vi "temperature sweep -- read log.vi"() -> ()   [LabVIEW 2010]
uses:
  <vilib>/Analysis/6fits.llb/Curve Fitting Criteria.ctl
  <vilib>/regexp/Match Regular Expression.xnode
  <vilib>/Utility/file.llb/Read From Spreadsheet File (string).vi
  <vilib>/Analysis/3filter.llb/IIR Filter (DBL).vi
  <vilib>/Analysis/NI_AALPro.lvlib
  <vilib>/ptbypt/NI_PtbyPt.lvlib
  <vilib>/Analysis/NI_AALBase.lvlib
panel:
  in  "window (min)":dbl=1.0
  out "window 5":cluster{dbl[], dbl[]}[](graph)
  out "window 4":cluster{dbl[], dbl[]}[](graph)
  out "window 3":cluster{dbl[], dbl[]}[](graph)
  out "window 2":cluster{dbl[], dbl[]}[](graph)
  out "window":cluster{dbl[], dbl[]}[](graph)
  in  "Control ITC Log":path=path "C:/Data/GloveBox/Pu/239 Pu A/300K - 600K/Stability_081211.dat"
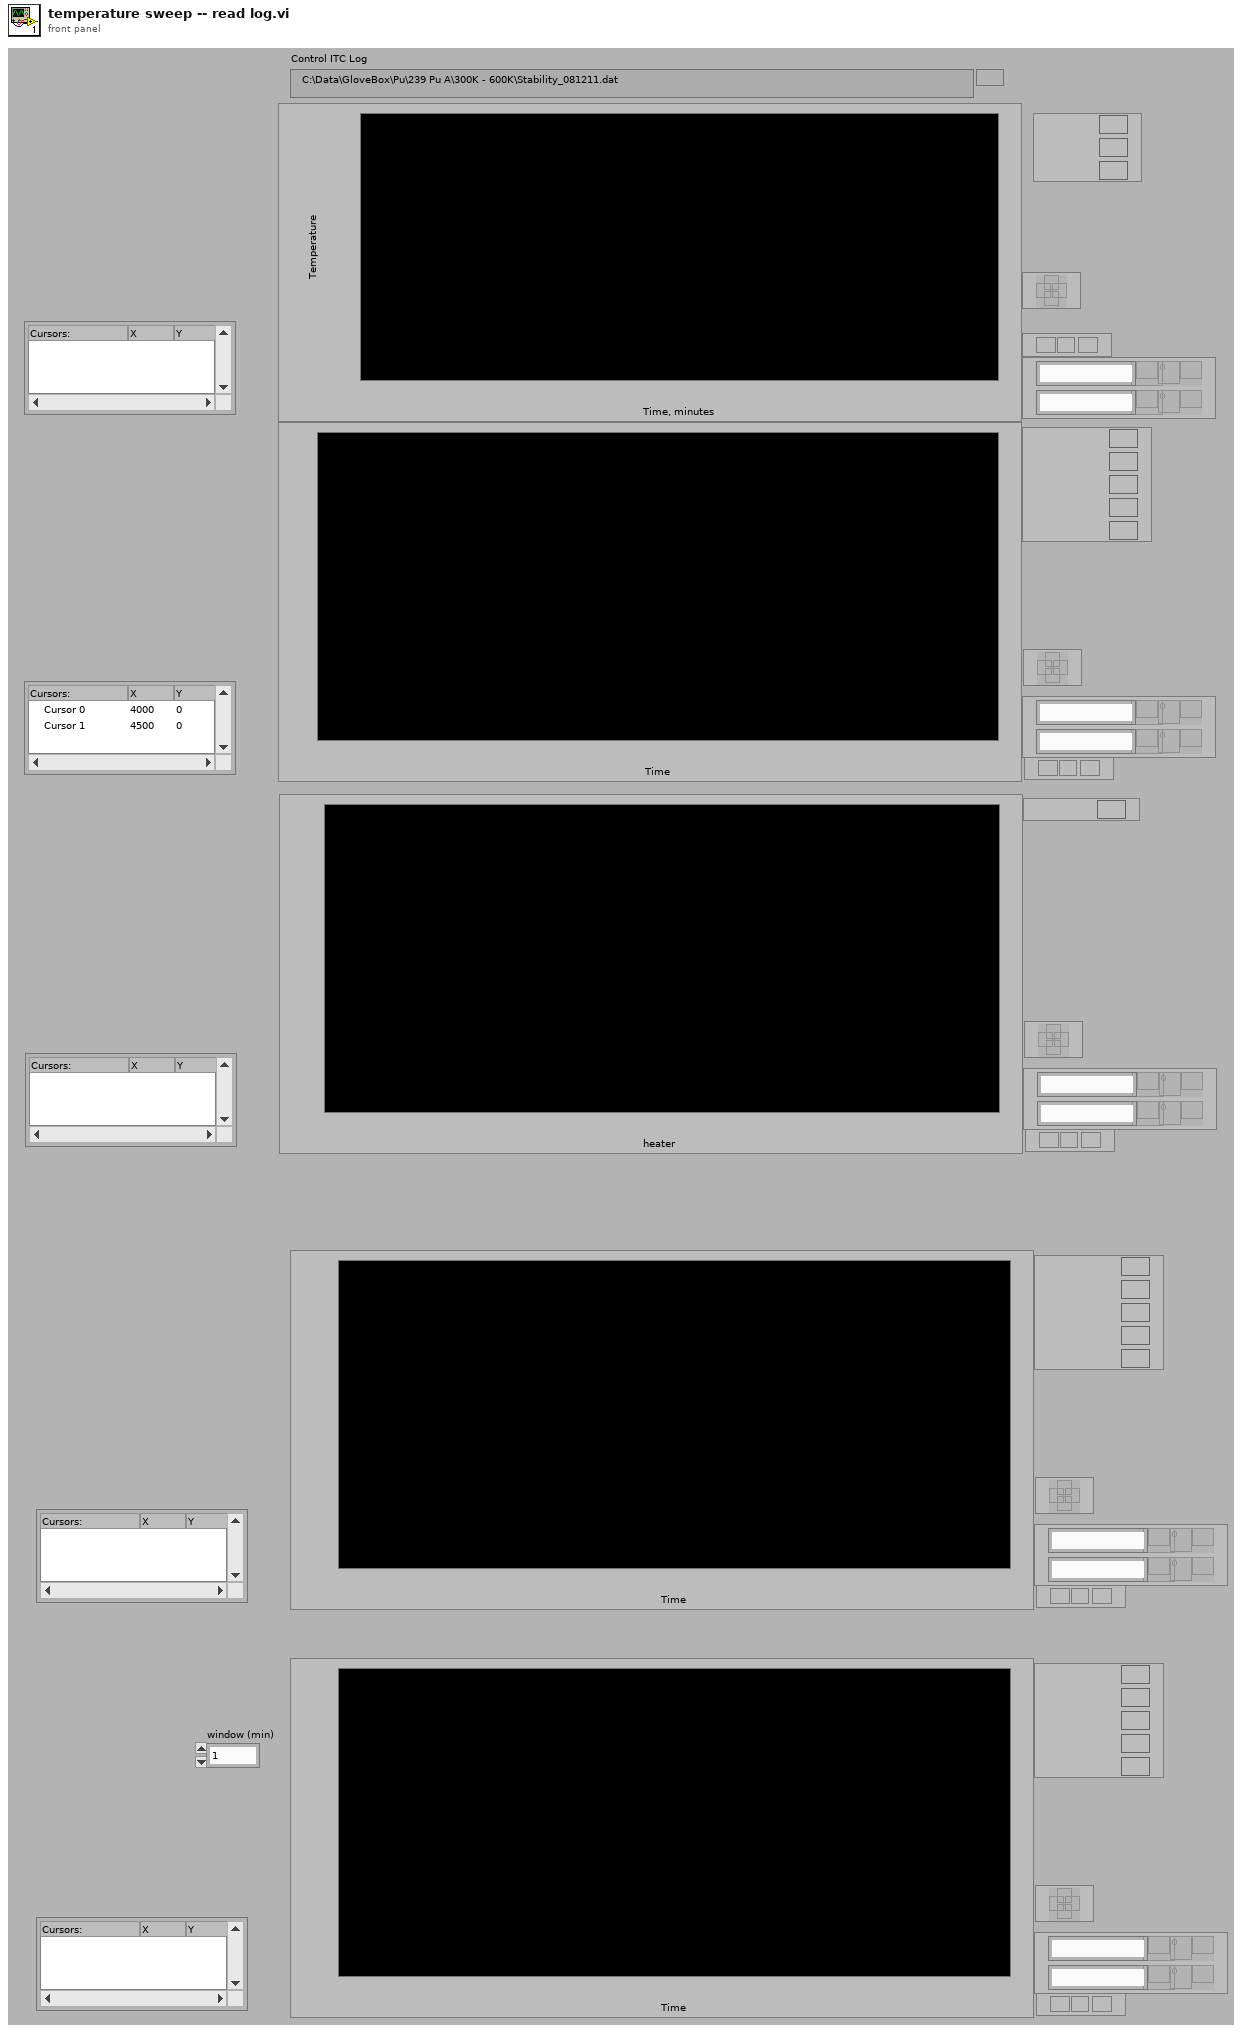
[diagram p1: front panel]
types:
  T1 = typedef "NI_AALPro.lvlib/Curve Fitting Criteria.ctl" = u16
  T2 = typedef "LVCursorListTypeDef.ctl" = cluster{"Name":string, "Color":u32, "Style":u8, "Point Style":u8, "Name Visible":bool, "Allow Drag":bool, "Cursor Mode":u32, "Plot":i32, "Index":i32, "Position":cluster{"X":dbl, "Y":dbl}, "X Scale":u32, "Y Scale":u32, "Watch Plots":i32[], "Watch All Plots":bool, "Plot Area":i32, "Label Offset":cluster{"X":dbl, "Y":dbl}}[]
  T3 = cluster{"omega out":dbl[], "whatever out":dbl[]}[]
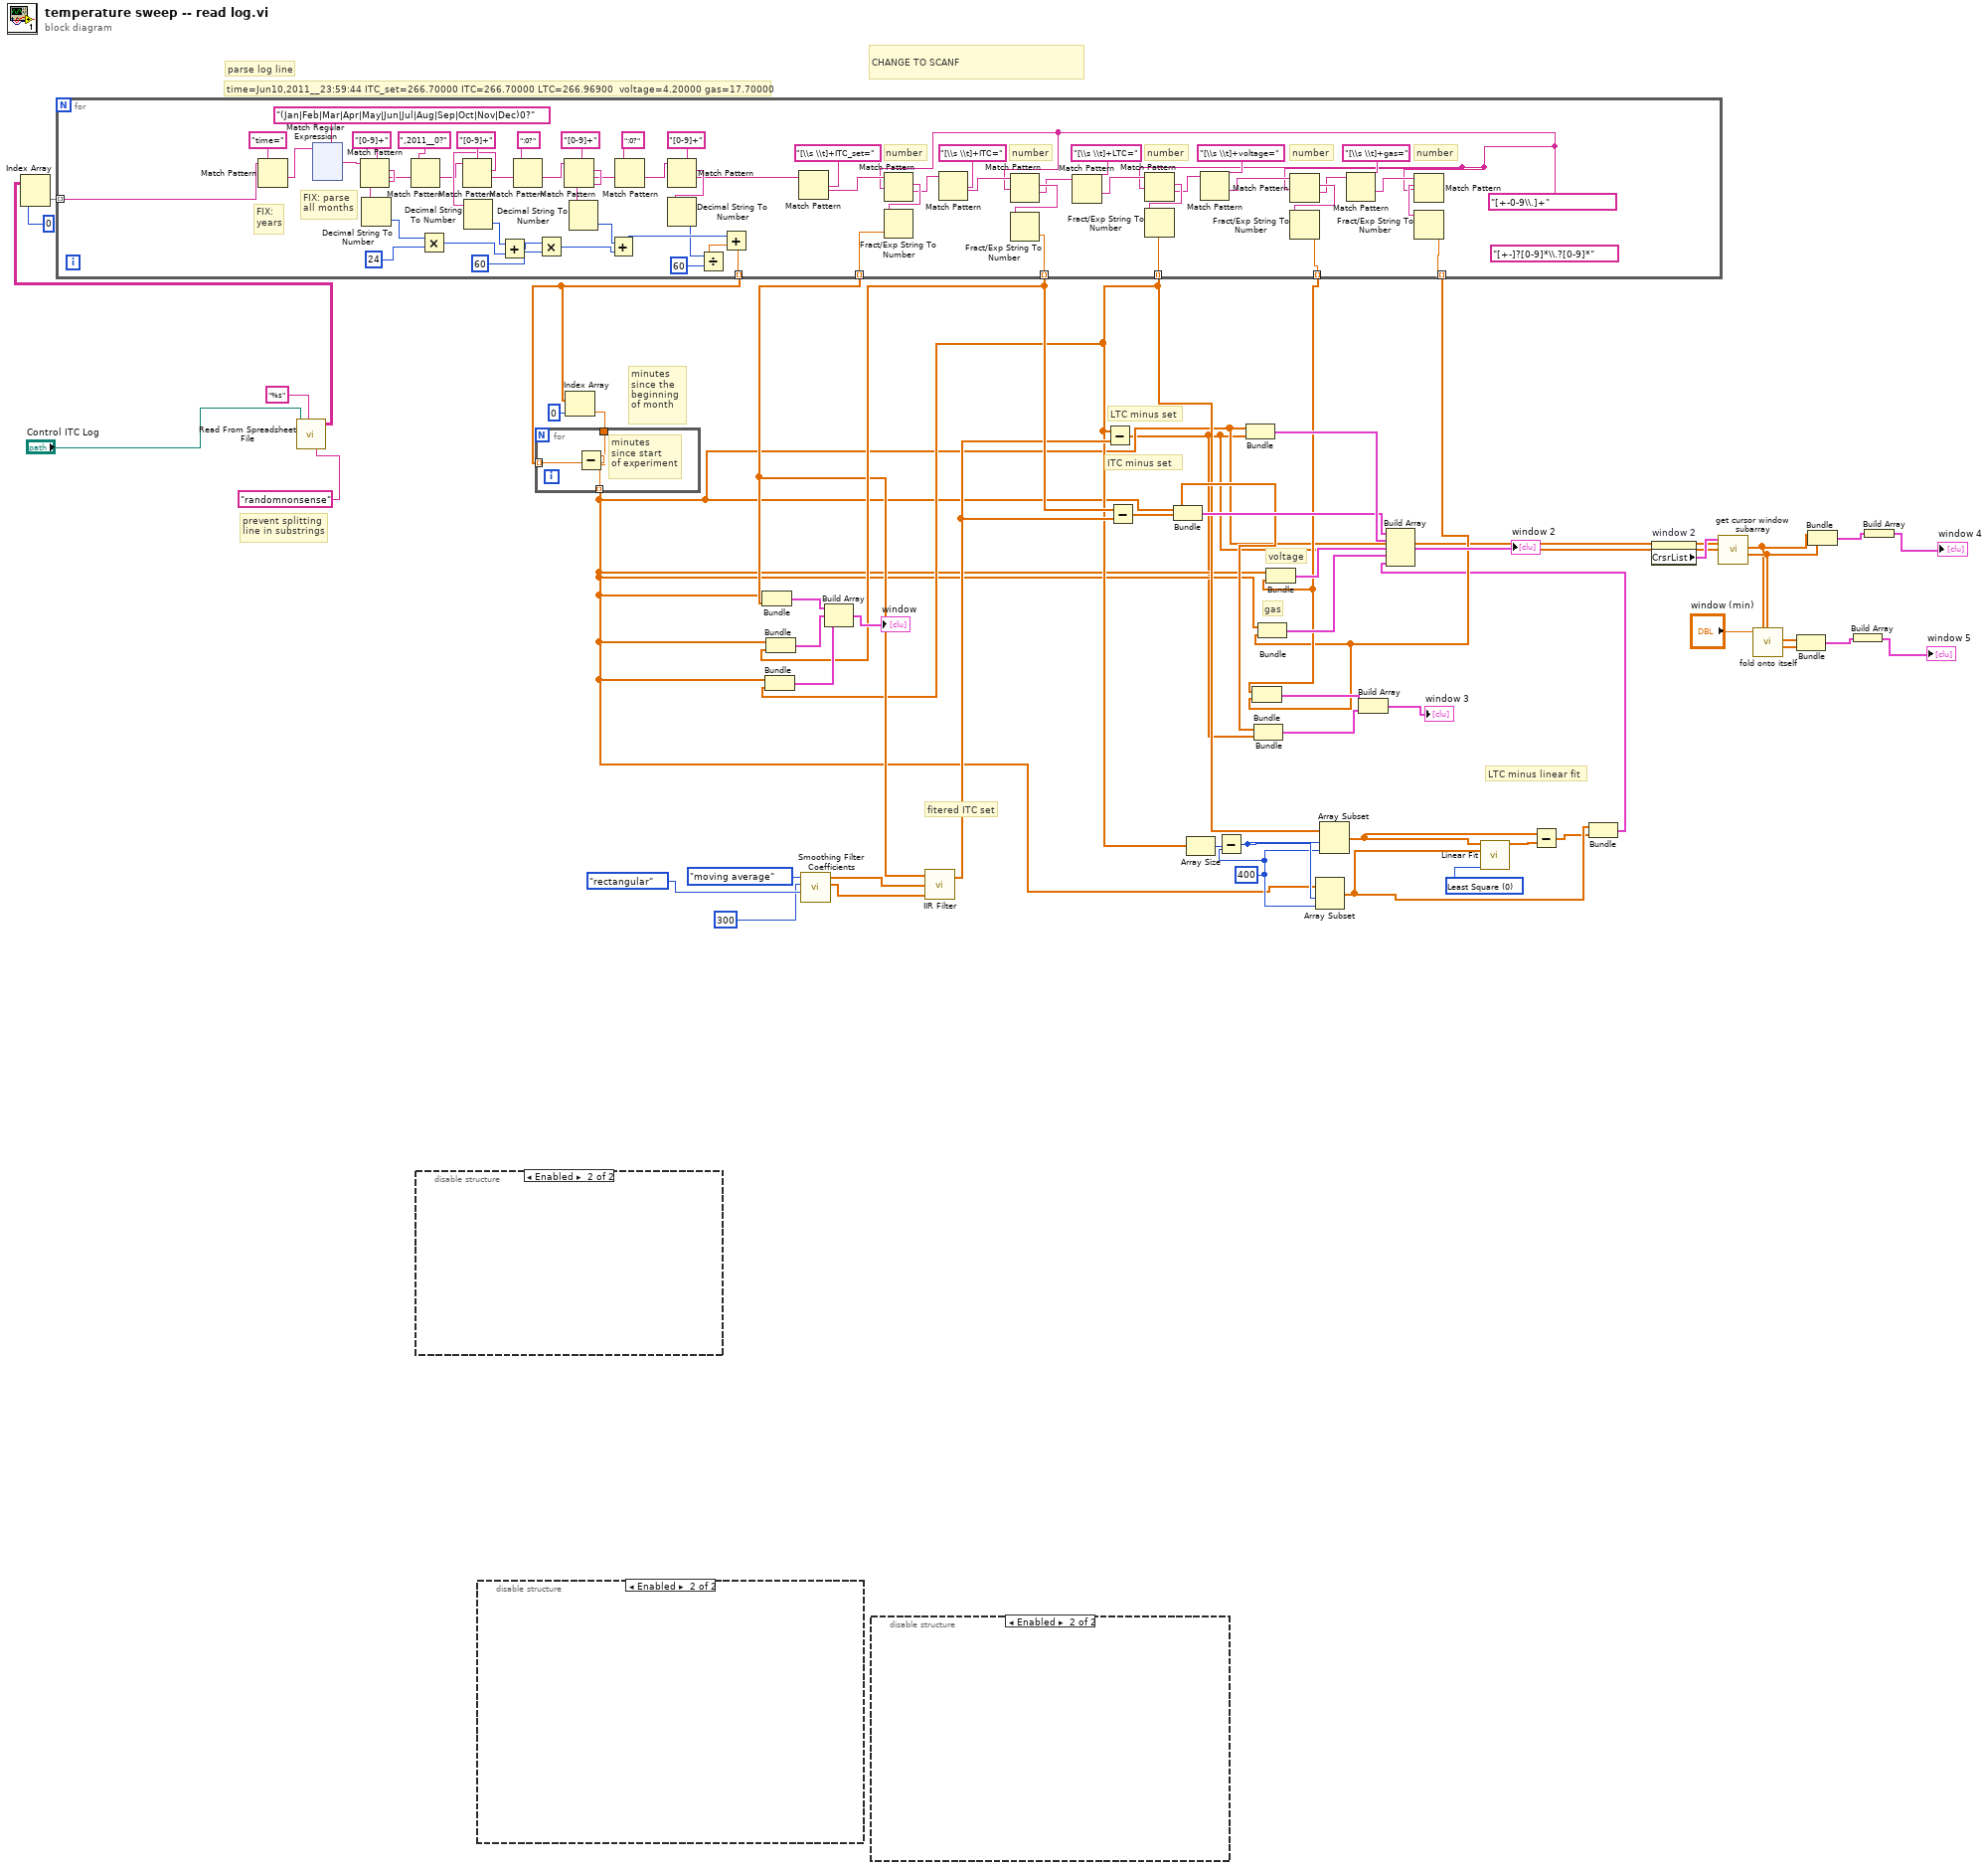
[diagram p0: block diagram]
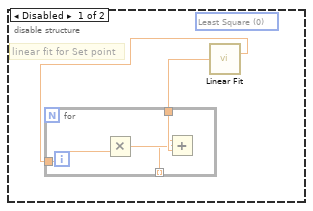
[diagram p2: hidden frame]
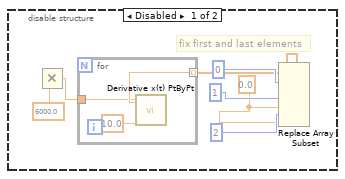
[diagram p3: hidden frame]
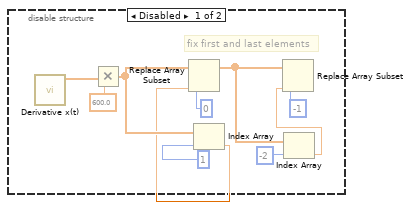
[diagram p4: hidden frame]
diagram:
  w18 = 400 ("length")
  w22 = T1 0 items=["Least Square", "Least Absolute Residual", "Bisquare"] ("method")
  # "fitered ITC set"
  # "CHANGE TO SCANF"
  # "LTC minus linear fit"
  # "minutes\nsince the\nbeginning \nof month"
  # "prevent splitting \nline in substrings"
  # "LTC minus set"
  # "gas"
  # "voltage"
  # "ITC minus set"
  # "parse log line"
  # "time=Jun10,2011__23:59:44\tITC_set=266.70000\tITC=266.70000\tLTC=266.96900\t\tvoltage=4.20000\tgas=17.70000"
  n1 = call-poly <vilib>:"Read From Spreadsheet File.vi"("delimiter (\\t)"="randomnonsense" ("delimiter (\\t)"), "format (%s)"="%s" ("format (%.3f)"), "file path (dialog if empty)"="Control ITC Log") -> ("all rows"=w51:string[][])  [unwired: 4 in, 4 out]
  n2 = Index Array(array=w51, index (col)=0 ("disabled index (col)")) -> (element=w43:string[])  [unwired: 1 in]
  n3 = for {
    tunnel: [w91] -> w31 mode=indexing
    tunnel: w43 -> [w86] mode=indexing
    tunnel: [w77] -> w29 mode=indexing
    tunnel: [w67] -> w30 mode=indexing
    tunnel: [w60] -> w21 mode=indexing
    tunnel: [w59] -> w37 mode=indexing
    tunnel: [w58] -> w32 mode=indexing
    w56 = "[+-0-9\\.]+" ("regular expression")
    (unwired) "[+-]?[0-9]*\\.?[0-9]*" ("regular expression")
    # "FIX:\nyears"
    # "FIX: parse \nall months"
    # "number"
    # "number"
    # "number"
    # "number"
    # "number"
    n4 = Match Pattern(string=w86, regular expression="time=") -> (after substring=w55:string)  [unwired: 1 in, 3 out]
    n5 = xnode "Match Regular Expression"("input string"=w55, "regular expression"="(Jan|Feb|Mar|Apr|May|Jun|Jul|Aug|Sep|Oct|Nov|Dec)0?") -> ("after match"=w113:string)  [unwired: 4 in, 4 out]
    n6 = Match Pattern(string=w113, regular expression="[0-9]+") -> (match substring=w111:string, after substring=w109:string)  [unwired: 1 in, 2 out]
    n7 = Decimal String To Number(string=w111) -> (number=w98:i32)  [unwired: 2 in, 1 out]
    n8 = Match Pattern(string=w109, regular expression=",2011__0?") -> (after substring=w93:string)  [unwired: 1 in, 3 out]
    n9 = Multiply(x=w98, y=24) -> (x*y=w84:i32)
    n10 = Match Pattern(string=w93, regular expression="[0-9]+") -> (match substring=w107:string, after substring=w105:string)  [unwired: 1 in, 2 out]
    n11 = Decimal String To Number(string=w107) -> (number=w85:i32)  [unwired: 2 in, 1 out]
    n12 = Add(x=w85, y=w84) -> (x+y=w95:i32)
    n13 = Match Pattern(string=w105, regular expression=":0?") -> (after substring=w94:string)  [unwired: 1 in, 3 out]
    n14 = Multiply(x=w95, y=60) -> (x*y=w83:i32)
    n15 = Match Pattern(string=w94, regular expression="[0-9]+") -> (match substring=w103:string, after substring=w101:string)  [unwired: 1 in, 2 out]
    n16 = Decimal String To Number(string=w103) -> (number=w82:i32)  [unwired: 2 in, 1 out]
    n17 = Add(x=w82, y=w83) -> (x+y=w90:i32)
    n18 = Match Pattern(string=w101, regular expression=":0?") -> (after substring=w92:string)  [unwired: 1 in, 3 out]
    n19 = Match Pattern(string=w92, regular expression="[0-9]+") -> (match substring=w99:string, after substring=w79:string)  [unwired: 1 in, 2 out]
    n20 = Decimal String To Number(string=w99) -> (number=w88:i32)  [unwired: 2 in, 1 out]
    n21 = Divide(x=w88, y=60) -> (x/y=w89:dbl)
    n22 = Add(x=w90, y=w89) -> (x+y=w91:dbl)
    n23 = Match Pattern(string=w79, regular expression="[\\s \\t]+ITC_set=") -> (after substring=w80:string)  [unwired: 1 in, 3 out]
    n24 = Match Pattern(string=w80, regular expression=w56) -> (match substring=w78:string, after substring=w68:string)  [unwired: 1 in, 2 out]
    n25 = Fract/Exp String To Number(string=w78) -> (number=w77:dbl)  [unwired: 3 in, 1 out]
    n26 = Match Pattern(string=w68, regular expression="[\\s \\t]+ITC=") -> (after substring=w76:string)  [unwired: 1 in, 3 out]
    n27 = Match Pattern(string=w76, regular expression=w56) -> (match substring=w75:string, after substring=w63:string)  [unwired: 1 in, 2 out]
    n28 = Fract/Exp String To Number(string=w75) -> (number=w67:dbl)  [unwired: 3 in, 1 out]
    n29 = Match Pattern(string=w63, regular expression="[\\s \\t]+LTC=") -> (after substring=w73:string)  [unwired: 1 in, 3 out]
    n30 = Match Pattern(string=w73, regular expression=w56) -> (match substring=w72:string, after substring=w62:string)  [unwired: 1 in, 2 out]
    n31 = Fract/Exp String To Number(string=w72) -> (number=w60:dbl)  [unwired: 3 in, 1 out]
    n32 = Match Pattern(string=w62, regular expression="[\\s \\t]+voltage=") -> (after substring=w70:string)  [unwired: 1 in, 3 out]
    n33 = Match Pattern(string=w70, regular expression=w56) -> (match substring=w69:string, after substring=w61:string)  [unwired: 1 in, 2 out]
    n34 = Fract/Exp String To Number(string=w69) -> (number=w59:dbl)  [unwired: 3 in, 1 out]
    n35 = Match Pattern(string=w61, regular expression="[\\s \\t]+gas=") -> (after substring=w65:string)  [unwired: 1 in, 3 out]
    n36 = Match Pattern(string=w65, regular expression=w56) -> (match substring=w64:string)  [unwired: 1 in, 3 out]
    n37 = Fract/Exp String To Number(string=w64) -> (number=w58:dbl)  [unwired: 3 in, 1 out]
  }
  n38 = disable-structure shown="Enabled" {
    frame Disabled {
      (unwired) T1 0 items=["Least Square", "Least Absolute Residual", "Bisquare"] ("method")
      # "linear fit for Set point"
      n39 = call <vilib>:"Linear Fit.vi"() -> ("slope"=w227:dbl, "intercept"=w228:dbl, "method"=w229:T1)  [unwired: 10 in, 3 out]
      n40 = for {
        tunnel: w228 -> [w233]
        tunnel: w227 -> [w232]
        tunnel: [w230] -> _ mode=indexing
        n41 = Multiply(y=w232) -> (x*y=w231:dbl)  [unwired: 1 in]
        n42 = Add(x=w231, y=w233) -> (x+y=w230:dbl)
      }
    }
    frame Enabled {
    }
  }
  n43 = disable-structure shown="Enabled" {
    frame Disabled {
      # "fix first and last elements"
      n44 = call <vilib>:"Derivative x(t).vi"() -> ("dX/dt"=w243:dbl[])  [unwired: 10 in, 1 out]
      n45 = Multiply(x=w243, y=600.0) -> (x*y=w241:dbl[])
      n46 = Index Array(array=w241, index=1) -> (element=w239:dbl)
      n47 = Replace Array Subset(array=w241, new element=w239, index=0) -> (w235:dbl[])
      n48 = Index Array(array=w235, index=-2) -> (element=w237:dbl)
      n49 = Replace Array Subset(array=w235, new element=w237, index=-1) -> (w234:dbl[])
    }
    frame Enabled {
    }
  }
  n50 = Index Array(array=w31, index=0) -> (element=w39:dbl)
  n51 = for {
    tunnel: w31 -> [w247] mode=indexing
    tunnel: w39 -> [w246]
    tunnel: [w245] -> w9 mode=indexing
    # "minutes\nsince start \nof experiment"
    n52 = Subtract(x=w247, y=w246) -> (x-y=w245:dbl)
  }
  n53 = Bundle(w9, w29) -> (w49:cluster{dbl[], dbl[]})  [unwired: 1 in]
  n54 = Bundle(w9, w21) -> (w47:cluster{dbl[], dbl[]})  [unwired: 1 in]
  n55 = Bundle(w9, w30) -> (w48:cluster{dbl[], dbl[]})  [unwired: 1 in]
  n56 = call <vilib>:"Smoothing Filter Coefficients.vi"("shape"=enum16{"rectangular", "triangular"}."rectangular", "half-width"=300, "type"=enum16{"moving average", "exponential"}."moving average") -> ("forward coefficients"=w26:dbl[], "reverse coefficients"=w27:dbl[])  [unwired: 6 in, 1 out]
  n57 = Build Array(w49, w48, w47) -> (→"window":cluster{dbl[], dbl[]}[])
  n58 = disable-structure shown="Enabled" {
    frame Disabled {
      w250 = 0.0 ("new element/subarray")
      # "fix first and last elements"
      n59 = Multiply(y=6000.0) -> (x*y=w254:dbl)  [unwired: 1 in]
      n60 = for {
        tunnel: [w258] -> w249 mode=indexing
        tunnel: w254 -> [w257]
        n61 = call <vilib>:"Derivative x(t) PtByPt.vi"("dt"=10.0, "x"=w257) -> ("dx/dt"=w258:dbl)  [unwired: 2 in, 1 out]
      }
      n62 = Replace Array Subset(array=w249, new element #1=w250, index #1=0 ("index"), new element #2=w250, index #2=1 ("index"), new element #3=w250, index #3=2 ("index")) -> (w248:dbl[])
    }
    frame Enabled {
    }
  }
  n63 = call-poly <vilib>:"IIR Filter.vi"("Forward Coefficients"=w26, "Reverse Coefficients"=w27, "X"=w29) -> ("Filtered X"=w28:dbl[])  [unwired: 1 in, 1 out]
  n64 = Subtract(x=w21, y=w28) -> (x-y=w8:dbl[])
  n65 = Subtract(x=w30, y=w28) -> (x-y=w34:dbl[])
  n66 = Bundle(w9, w34) -> (w41:cluster{dbl[], dbl[]})  [unwired: 1 in]
  n67 = Array Size(array=w21) -> (size(s)=w20:i32)
  n68 = Subtract(x=w20, y=w18) -> (x-y=w19:i32)
  n69 = Bundle(w9, w8) -> (w42:cluster{dbl[], dbl[]})  [unwired: 1 in]
  n70 = Bundle(w37, w32) -> (w35:cluster{dbl[], dbl[]})  [unwired: 1 in]
  n71 = Bundle(w34, w8) -> (w33:cluster{dbl[], dbl[]})  [unwired: 1 in]
  n72 = Bundle(w9, w32) -> (w44:cluster{dbl[], dbl[]})  [unwired: 1 in]
  n73 = Bundle(w9, w37) -> (w45:cluster{dbl[], dbl[]})  [unwired: 1 in]
  n74 = Array Subset(array=w9, index=w19, length=w18) -> (w13:dbl[])
  n75 = Array Subset(array=w21, index=w19, length=w18) -> (w17:dbl[])
  n76 = Build Array(w35, w33) -> (→"window 3":cluster{dbl[], dbl[]}[])
  n77 = call <vilib>:"Linear Fit.vi"("Y"=w17, "X"=w13, "method"=w22) -> ("Best Linear Fit"=w16:dbl[])  [unwired: 8 in, 4 out]
  n78 = Subtract(x=w17, y=w16) -> (x-y=w12:dbl[])
  n79 = Bundle(w13, w12) -> (w15:cluster{dbl[], dbl[]})  [unwired: 1 in]
  n80 = Build Array(w41, w42, w45, w44, w15) -> (→"window 2":cluster{dbl[], dbl[]}[])
  n81 = property on="window 2" class="XYGraph (strict)"() -> ("CrsrList"=w14:T2)  [unwired: 2 in, 2 out]
  n82 = call "get cursor window subarray.vi"("whatever"=w8, "omega"=w9, "Cursor List"=w14) -> ("whatever out"=w3:dbl[], "omega out"=w2:dbl[])  [unwired: 7 in]
  n83 = call "fold onto itself.vi"("whatever"=w3, "omega"=w2, "window size"="window (min)") -> ("whatever out"=w4:dbl[], "omega out"=w5:dbl[])  [unwired: 7 in]
  n84 = Bundle("omega out"=w5, "whatever out"=w4) -> (w7:cluster{"omega out":dbl[], "whatever out":dbl[]})  [unwired: 1 in]
  n85 = Bundle("omega out"=w2, "whatever out"=w3) -> (w11:cluster{"omega out":dbl[], "whatever out":dbl[]})  [unwired: 1 in]
  n86 = Build Array(w7) -> (→"window 5":T3)
  n87 = Build Array(w11) -> (→"window 4":T3)
